vi "Graph_REQUEST_DATA_to_SERVER.vi"(7 "Control Name":string="MOKO_STAGE", 8 "Error In":errorcluster, 11 "MOKO_Graph_STM":T1={"main stm"=enum."idle", "data"="{Hello world!}"}) -> (0 "Error Out":errorcluster)   [LabVIEW 2018]
uses:
  STM/Graph/MOKO_Graph_main_STM.ctl
  STM/Graph/MOKO_Graph_main_ITEM.ctl
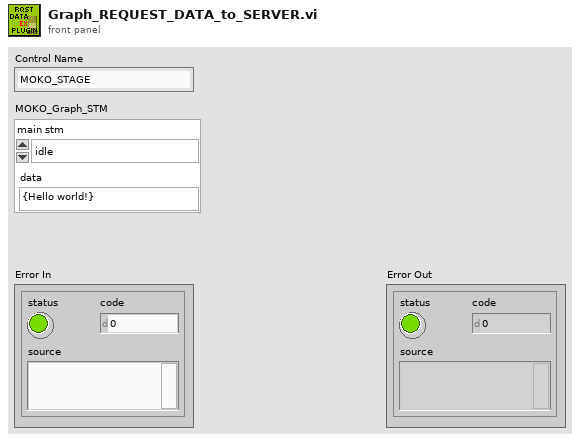
[diagram p1: front panel]
types:
  T1 = typedef "MOKO_Graph_main_STM.ctl" = cluster{"main stm":T2, "data":string}
  T2 = typedef "MOKO_Graph_main_ITEM.ctl" = enum16{"idle", "Graph read", "Graph write"}
  T3 = enum32{"Invalid", "Default", "Floating", "Floating/Auto-Hide", "Modal"}
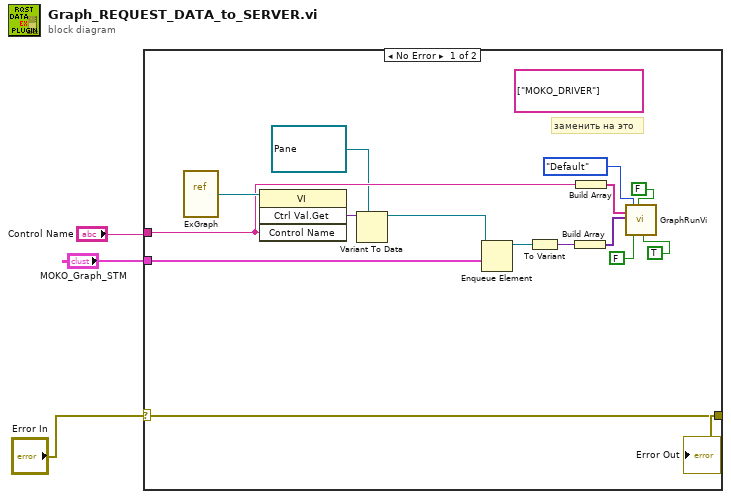
[diagram p0: block diagram]
diagram:
  n1 = case shown="No Error" "Error In" {
    selector: "Error In" -> [w14 w20]
    tunnel: [w14 w20] -> w3
    tunnel: "MOKO_Graph_STM" -> [w13 _]
    tunnel: "Control Name" -> [w12 _]
    frame No Error {
      (unwired) string[] ["MOKO_DRIVER"] ("Controls Name")
      # "заменить на это"
      n2 = vi-ref "ExGraph.vi"() -> (w17:refnum<vi>)
      n3 = invoke class="VI" method="Ctrl Val.Get"(reference=w17, "Control Name"=w12) -> ("Get Control Value Variant"=w18:variant)  [unwired: 2 in, 3 out]
      n4 = Variant To Data(type=refnum<queue> refnum ("MOKO_NMEA"), Variant=w18) -> (data=w19:refnum<queue>)  [unwired: 1 in, 1 out]
      n5 = Enqueue Element(queue=w19, element=w13) -> (queue out=w16:refnum<queue>)  [unwired: 2 in, 2 out]
      n6 = To Variant(anything=w16) -> (Variant=w15:variant)
      n7 = Build Array(w15) -> (w9:variant[])
      n8 = Build Array(w12) -> (w10:string[])
      n9 = call "GraphRunVi.vi"("Controls Name"=w10, "Values"=w9, "Front Panel Behavior"=T3."Default", "Wait Until Done"=FALSE, "ShowFP"=FALSE, "DoNotCentered If RUN"=TRUE) -> ()  [unwired: 13 in, 1 out]
    }
    frame Error {
    }
  }
  "Error Out" <- w3
